vi "GetScreenCap.vi"(8 "error in (no error)":errorcluster, 11 "Win Name":string) -> (0 "error out":errorcluster, 3 "Image Out":T1)   [LabVIEW 2025]
uses:
  <vilib>/vision/Image Controls.llb/IMAQ Image.ctl
  aa95d816-2e2f-41ff-8d1d-06727f7bfeb0.vi
  83e2a9eb-5231-41f3-a798-ce33e3325a13.vi
  <vilib>/Utility/error.llb/Trim Whitespace One-Sided.vi
  user32.dll
  <vilib>/vision/NI_Vision_Development_Module.lvlib
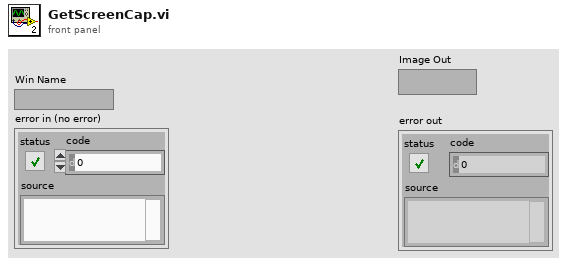
[diagram p1: front panel]
types:
  T1 = typedef "IMAQ Image.ctl" = refnum<image>
  T2 = enum16{"Left Mouse Button", "Right Mouse Button", "Ctrl-Break", "Middle Mouse Button (3-button mice only)", "X1 mouse button (Win2k Only)", "X2 Mouse Button (Win2k Only)", "Undefined (1)", "BACKSPACE", "TAB", "Reserved (1)", "Reserved (2)", "CLEAR", "ENTER", "Undefined (2)", "Undefined (3)", "SHIFT", "CTRL", "ALT", "PAUSE", "CAPS LOCK", "IME Kana mode", "Undefined (4)", "IME Junja mode", "IME final mode", "IME Hanja mode", "IME Kanji mode", "Undefined    ", "ESC", "IME convert", "IME nonconvert", "IME accept", "IME mode change request", "SPACEBAR", "PAGE UP", "PAGE DOWN", "END", "HOME", "LEFT ARROW", "UP ARROW", "RIGHT ARROW", "DOWN ARROW", "SELECT", "PRINT", "EXECUTE", "PRINT SCREEN", "INS", "DEL", "HELP"}
  T3 = typedef "Image Type" = u32
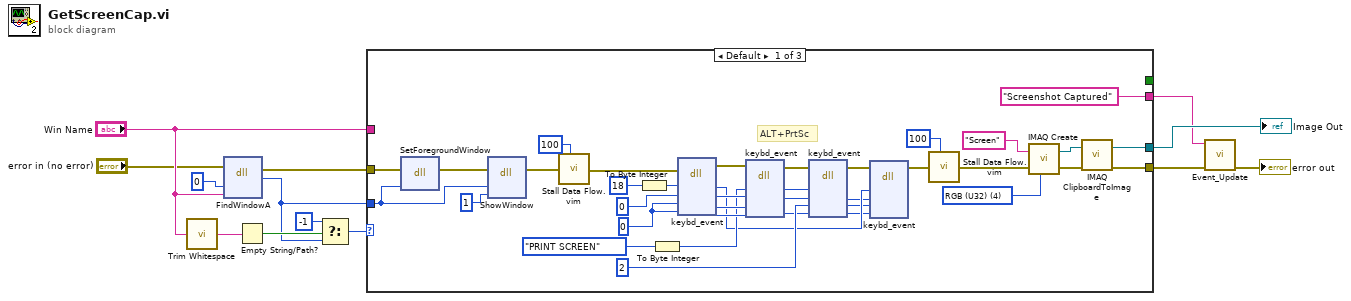
[diagram p0: block diagram]
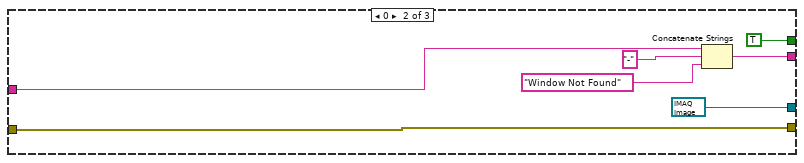
[diagram p2: hidden frame]
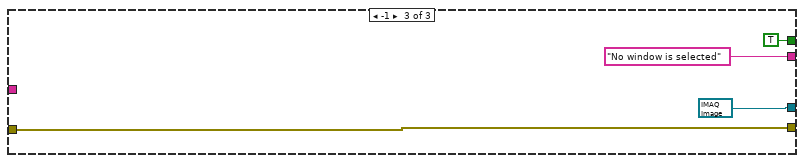
[diagram p3: hidden frame]
diagram:
  n1 = call <vilib>:"Trim Whitespace.vi"("string"="Win Name") -> ("trimmed string"=w11:string)  [unwired: 1 in]
  n2 = dll-call lib="user32.dll" fn="FindWindowA"(error in="error in (no error)", "arg1"=0, "arg2"="Win Name") -> (error out=w12:errorcluster, "return type"=w9:i32)  [unwired: 3 in, 2 out]
  n3 = Empty String/Path?(string/path=w11) -> (empty?=w10:bool)
  n4 = Select(t=-1, s=w10, f=w9) -> (s? t:f=w7:i32)
  n5 = case shown="Default" w7 {
    tunnel: "Win Name" -> [_ w57 _]
    tunnel: [w45 w53 w61] -> w3
    tunnel: ["Screenshot Captured" w54 "No window is selected"] -> w1
    tunnel: w9 -> [w43 _ _]
    tunnel: w12 -> [w44 w53 w61]
    tunnel: [w15 T1 refnum ("Image Out") T1 refnum ("Image Out")] -> w4
    tunnel: [_ TRUE ("Error?") TRUE ("Error?")] -> _
    frame Default {
      w18 = T3 4 items=["Grayscale (U8)", "Grayscale (I16)", "Grayscale (SGL)", "Complex (CSG)", "RGB (U32)", "HSL (U32)", "RGB (U64)", "Grayscale (U16)"] ("Image Type")
      w41 = 0 ("Input Value")
      # "ALT+PrtSc"
      n6 = dll-call lib="user32.dll" fn="SetForegroundWindow"(error in=w44, "arg1"=w43) -> (error out=w48:errorcluster)  [unwired: 3 in, 2 out]
      n7 = dll-call lib="user32.dll" fn="ShowWindow"(error in=w48, "arg1"=w43, "arg2"=1) -> (error out=w47:errorcluster)  [unwired: 4 in, 2 out]
      n8 = call "Stall Data Flow.vim"("value in"=w47, "milliseconds to wait"=u32 100) -> ("value out"=w50:errorcluster)  [unwired: 1 out]
      n9 = To Byte Integer(number=i8 18) -> (8bit integer=w22:i8)
      n10 = To Byte Integer(number=T2."PRINT SCREEN" ("Keyboard Stroke")) -> (8bit integer=w32:i8)
      n11 = dll-call lib="user32.dll" fn="keybd_event"(error in=w50, w22, i8 0, w41, w41) -> (error out=w39:errorcluster, w27:i8, w36:i8, w35:i32, w34:i32)  [unwired: 3 in, 1 out]
      n12 = dll-call lib="user32.dll" fn="keybd_event"(error in=w39, w32, w36, w35, w34) -> (error out=w37:errorcluster, w31:i8, w30:i8, w28:i32)  [unwired: 4 in, 1 out]
      n13 = dll-call lib="user32.dll" fn="keybd_event"(error in=w37, w31, w30, 2, w28) -> (error out=w38:errorcluster, w26:i8, w25:i32, w24:i32)  [unwired: 4 in, 1 out]
      n14 = dll-call lib="user32.dll" fn="keybd_event"(error in=w38, w27, w26, w25, w24) -> (error out=w49:errorcluster)  [unwired: 7 in, 1 out]
      n15 = call "Stall Data Flow.vim"("value in"=w49, "milliseconds to wait"=u32 100) -> ("value out"=w17:errorcluster)  [unwired: 1 out]
      n16 = call "IMAQ Create"("Image Name"="Screen", "Image Type"=w18, "error in (no error)"=w17) -> ("New Image"=w19:T1, "error out"=w16:errorcluster)  [unwired: 2 in]
      n17 = call "IMAQ ClipboardToImage"("error in (no error)"=w16, "Image"=w19) -> ("error out"=w45:errorcluster, "Image Out"=w15:T1)  [unwired: 3 in, 2 out]
    }
    frame 0 {
      n18 = Concatenate Strings(w57, "-" ("string"), "Window Not Found") -> (w54:string)
    }
    frame -1 {
    }
  }
  "Image Out" <- w4
  n19 = call "Event_Update.vi"("Error In"=w3, "Event"=w1) -> ("Error Out"=→"error out":errorcluster)  [unwired: 9 in]
